vi "UDP数字量输出发送接收.vi"(8 "发送值":enum16{"0", "1"}(ring), 10 "第几组":i32) -> (0 "异常_找到?":bool, 1 "接收超时?":bool, 2 "接收的一帧数据":u16[](array[numeric]), 3 "正常_找到?":bool)   [LabVIEW 2010]
uses:
  全局量/全局_配置.vi
panel:
  out "开始时间":dbl format="%#.0f"
  # "从0开始"
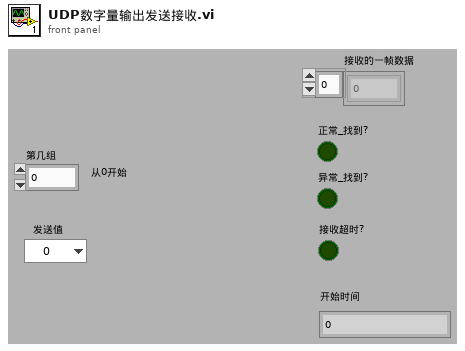
[diagram p1: front panel]
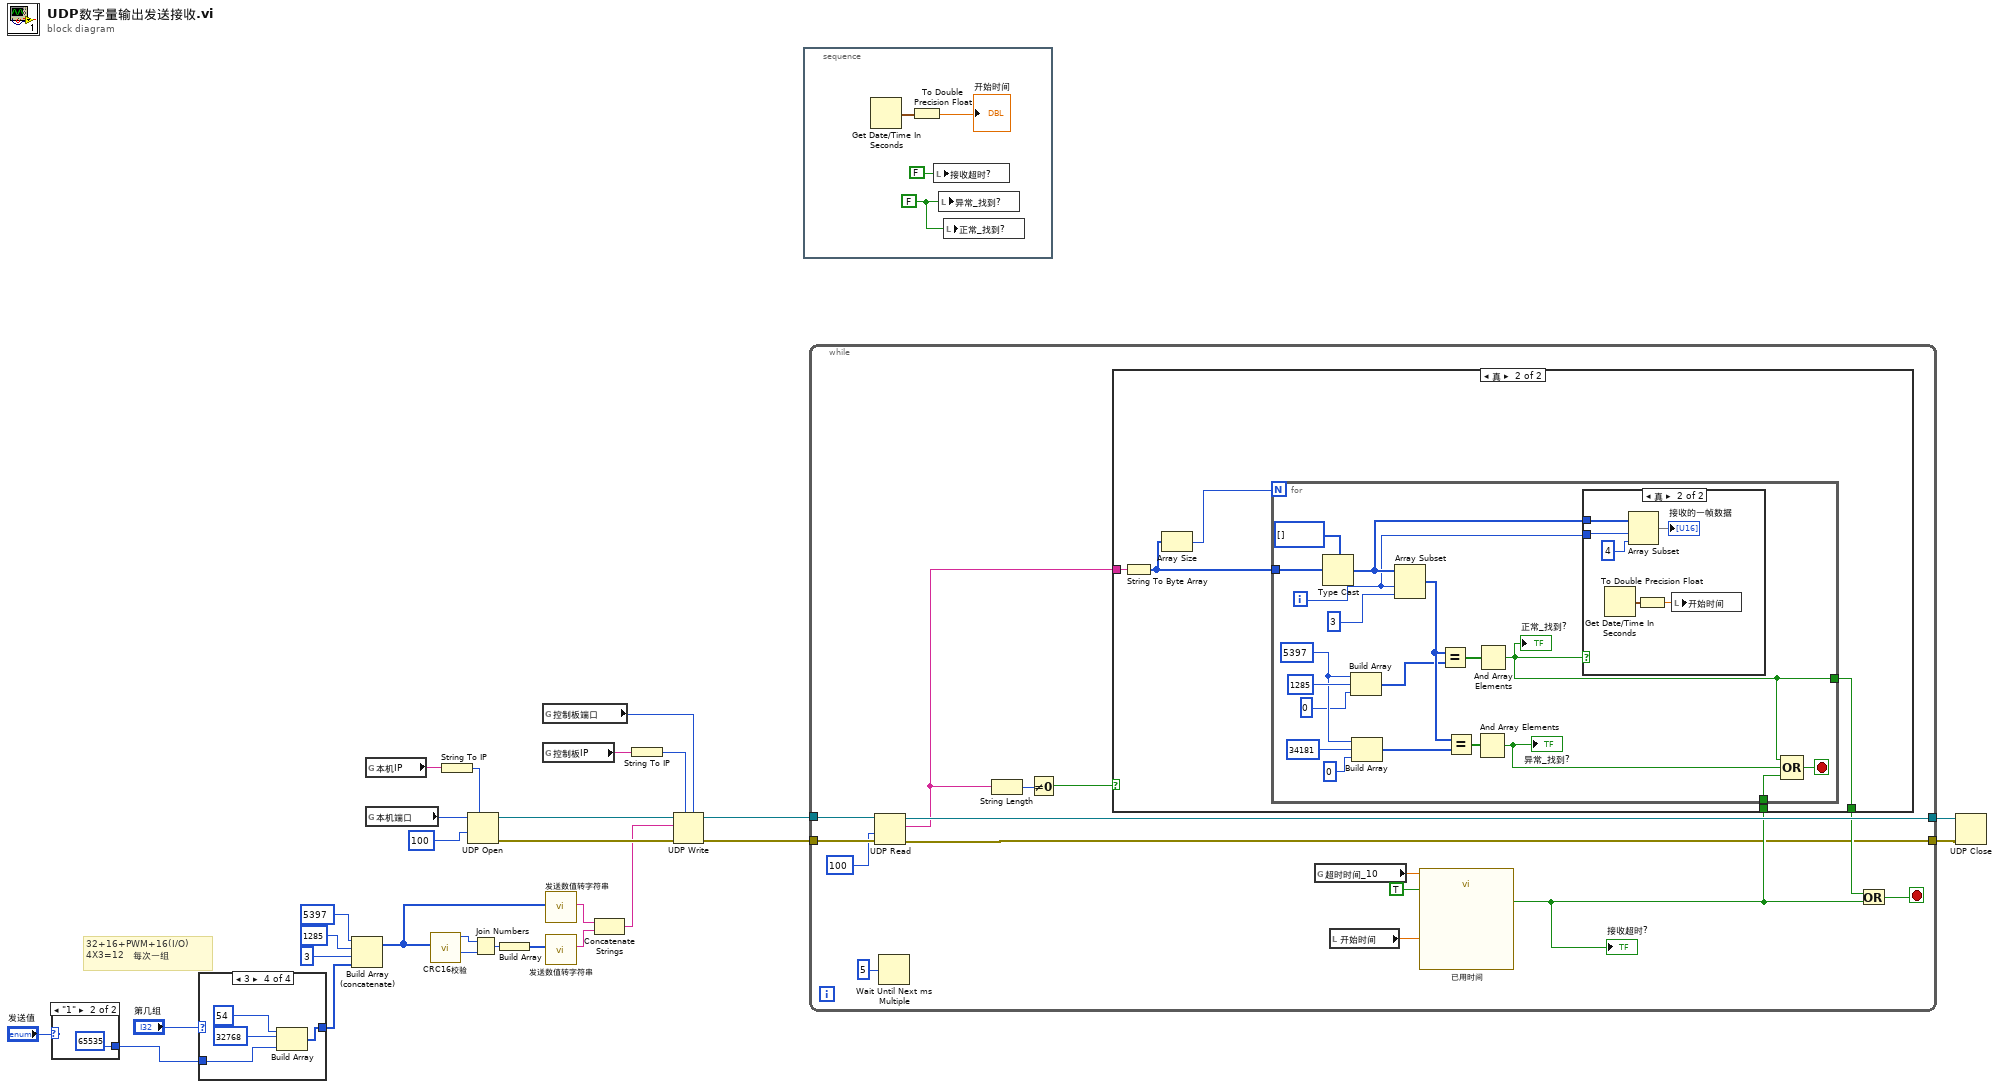
[diagram p0: block diagram]
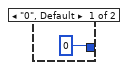
[diagram p2: hidden frame]
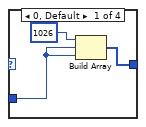
[diagram p3: hidden frame]
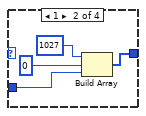
[diagram p4: hidden frame]
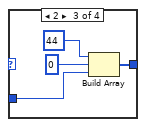
[diagram p5: hidden frame]
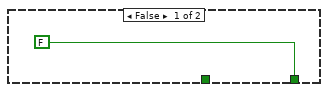
[diagram p6: hidden frame]
diagram:
  # "32+16+PWM+16(I/O)\n4X3=12   每次一组"
  n1 = case shown="\"1\"" "发送值" {
    tunnel: [u16 0 u16 65535] -> w2
    frame "0", Default {
    }
    frame "1" {
    }
  }
  n2 = case shown="3" "第几组" {
    tunnel: w2 -> [w32 w36 w39 w42]
    tunnel: [w31 w35 w38 w43] -> w1
    frame 0, Default {
      n3 = Build Array(u16 1026, w32, w32) -> (w31:u16[])
    }
    frame 1 {
      n4 = Build Array(u16 1027, u16 0 ("数值_U16_0"), w36) -> (w35:u16[])
    }
    frame 2 {
      n5 = Build Array(u16 44, u16 0 ("数值_U16_0"), w39) -> (w38:u16[])
    }
    frame 3 {
      n6 = Build Array(u16 54, u16 32768, w42) -> (w43:u16[])
    }
  }
  n7 = Build Array (concatenate)(u16 5397, u16 1285, u16 3, w1) -> (w22:u16[])
  n8 = global read "全局_配置.vi" "本机IP"() -> (w26:string)
  n9 = global read "全局_配置.vi" "本机端口"() -> (w24:u16)
  n10 = call "CRC16校验.vi"("输入数据_U16"=w22) -> ("低字节"=w17:u8, "高字节"=w16:u8)  [unwired: 9 in]
  n11 = String To IP(1:w26) -> (0:w25:u32)
  n12 = UDP Open(7:w25, 9:100 ("超时毫秒(25000)"), 11:w24) -> (port=w11:refnum<k16>, 0:w10:errorcluster)  [unwired: 2 in, 1 out]
  n13 = Join Numbers(hi=w16, lo=w17) -> ((hi.lo)=w20:u16)
  n14 = Build Array(w20) -> (w21:u16[])
  n15 = global read "全局_配置.vi" "控制板端口"() -> (w6:u16)
  n16 = global read "全局_配置.vi" "控制板IP"() -> (w12:string)
  n17 = call "发送数值转字符串.vi"("输入数据_U16"=w22) -> ("字符串"=w18:string)  [unwired: 10 in]
  n18 = call "发送数值转字符串.vi"("输入数据_U16"=w21) -> ("字符串"=w19:string)  [unwired: 10 in]
  n19 = Concatenate Strings(w18, w19) -> (w5:string)
  n20 = String To IP(1:w12) -> (0:w7:u32)
  n21 = UDP Write(address=w7, port or service name=w6, connection ID=w11, data in=w5, 8:w10) -> (error out=w8:errorcluster, 3:w9:refnum<k16>)  [unwired: 1 in]
  n22 = stacked-sequence {
    frame #0 {
      w47 = FALSE ("找到?")
      n23 = Get Date/Time In Seconds() -> (seconds since 1Jan1904=w49:timestamp)
      n24 = To Double Precision Float(number=w49) -> (double precision float=→"开始时间":dbl)
      n25 = local write "接收超时?"(FALSE ("接收超时?")) -> ()
      n26 = local write "异常_找到?"(w47) -> ()
      n27 = local write "正常_找到?"(w47) -> ()
    }
  }
  n28 = while {
    tunnel: w9 -> [w64]
    tunnel: w8 -> [w63]
    tunnel: [w62] -> w28
    tunnel: [w50] -> w27
    stop <- w54 stop-if-true
    n29 = UDP Read(connection ID=w64, timeout ms (25000)=100, 8:w63) -> (data out=w53:string, error out=w50:errorcluster, 3:w62:refnum<k16>)  [unwired: 1 in, 2 out]
    n30 = Wait Until Next ms Multiple(millisecond multiple=u32 5 ("毫秒倍数")) -> ()  [unwired: 1 out]
    n31 = String Length(string=w53) -> (length=w60:i32)
    n32 = Not Equal To 0?(x=w60) -> (x != 0?=w59:bool)
    n33 = global read "全局_配置.vi" "超时时间_10"() -> (w57:dbl)
    n34 = local read "开始时间"() -> (w56:dbl)
    n35 = call "已用时间"("Time Target (s)"=w57, "Reset"=TRUE, "Set Start Time (s)"=w56) -> ("Time has Elapsed"=w51:bool)  [unwired: 9 in, 7 out]
    "接收超时?" <- w51
    n36 = case shown="真" w59 {
      tunnel: w53 -> [_ w69]
      tunnel: [FALSE ("找到?") w70] -> w55
      tunnel: w51 -> [_ w68]
      frame False {
      }
      frame True {
        n37 = String To Byte Array(string=w69) -> (unsigned byte array=w67:u8[])
        n38 = Array Size(array=w67) -> (size(s)=w66:i32)
        n39 = for {
          N: w66 -> [_]
          tunnel: w67 -> [w89]
          tunnel: [w71] -> w70
          tunnel: w68 -> [w79]
          i -> [w82]
          stop <- w81 stop-if-true
          w77 = u16 5397
          n40 = Type Cast(type=u16[] [], x=w89) -> (*(type *) &x=w83:u16[])
          n41 = Build Array(w77, u16 1285, u16 0) -> (w73:u16[])
          n42 = Build Array(w77, u16 34181, u16 0 ("元素")) -> (w72:u16[])
          n43 = Array Subset(array=w83, index=w82, length=3 ("长度")) -> (w84:u16[])
          n44 = Equal?(x=w84, y=w73) -> (x = y?=w85:bool[])
          n45 = Equal?(x=w84, y=w72) -> (x = y?=w86:bool[])
          n46 = And Array Elements(Boolean array=w86) -> (logical AND=w80:bool)
          "异常_找到?" <- w80
          n47 = And Array Elements(Boolean array=w85) -> (logical AND=w71:bool)
          "正常_找到?" <- w71
          n48 = case shown="真" w71 {
            tunnel: w83 -> [_ w95]
            tunnel: w82 -> [_ w94]
            frame False {
            }
            frame True {
              n49 = Get Date/Time In Seconds() -> (seconds since 1Jan1904=w92:timestamp)
              n50 = Array Subset(array=w95, index=w94, length=4 ("长度")) -> (→"接收的一帧数据":u16[])
              n51 = To Double Precision Float(number=w92) -> (double precision float=w91:dbl)
              n52 = local write "开始时间"(w91) -> ()
            }
          }
          n53 = Compound Arithmetic op=OR(w71, w80, w79) -> (w81:bool)
        }
      }
    }
    n54 = Or(x=w55, y=w51) -> (x .or. y?=w54:bool)
  }
  n55 = UDP Close(connection ID=w28, 8:w27) -> ()  [unwired: 2 out]
